vi "Telnet_test.vi"(5 "report_path":path, 6 "bytes to read (1024)":i32=1024, 7 "Delay Time (s)":dbl=0.3, 8 "error in (no error)":errorcluster, 9 "expected string":string, 10 "Command":string) -> (0 "error out":errorcluster, 1 "String found?":bool, 2 "string out":string caption="string ou", 3 "connection ID out":refnum<k5>)   [LabVIEW 2018]
doc: "This VI sends a command using telnet and verifies the response is the expected one."
panel:
  out "Get challenge status":string
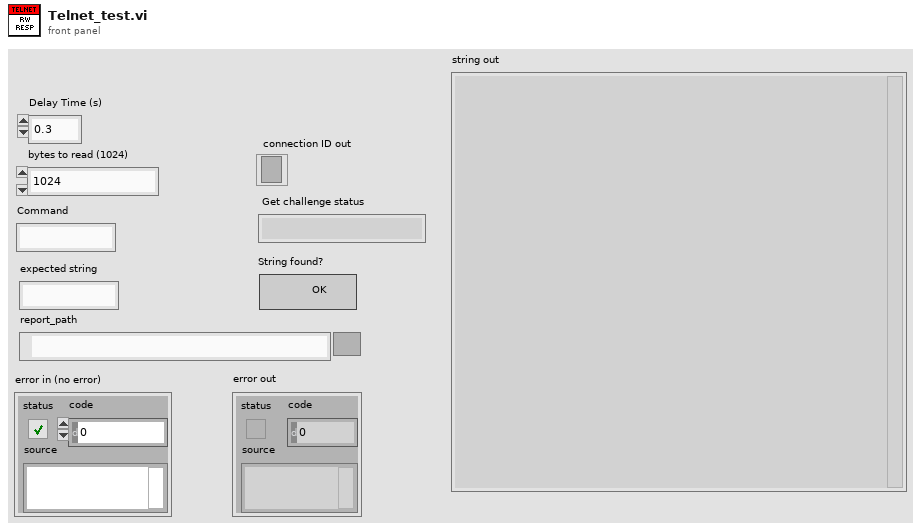
[diagram p1: front panel]
types:
  T1 = enum16{"Standard", "Buffered", "CRLF", "Immediate"}
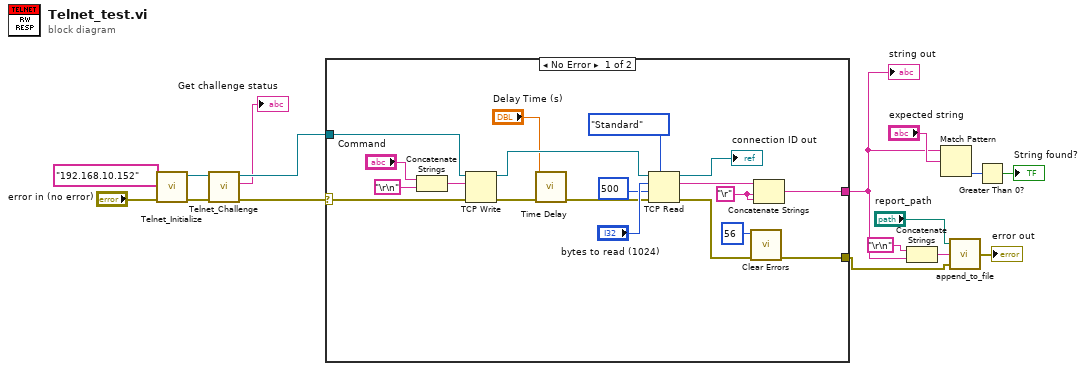
[diagram p0: block diagram]
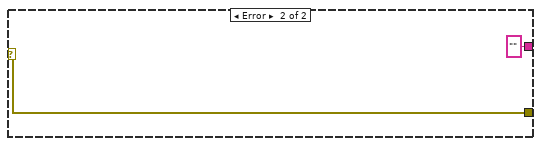
[diagram p2: hidden frame]
diagram:
  n1 = call "Telnet_Initialize.vi"("error in (no error)"="error in (no error)", "Address"="192.168.10.152") -> ("error out"=w5:errorcluster, "connection ID out"=w4:refnum<k5>)  [unwired: 8 in]
  n2 = call "Telnet_Challenge.vi"("error in (no error)"=w5, "connection ID in"=w4) -> ("error out"=w1:errorcluster, "Challenge status"=→"Get challenge status":string, "connection ID out"=w3:refnum<k5>)  [unwired: 7 in]
  n3 = case shown="No Error" w1 {
    selector: w1 -> [w19 w36]
    tunnel: [w26 ""] -> w9
    tunnel: [w25 w36] -> w8
    tunnel: w3 -> [w20 _]
    frame No Error {
      w27 = "\r"
      n4 = Concatenate Strings("Command", "\r\n") -> (w24:string)
      n5 = TCP Write(connection ID=w20, data in=w24, error in (no error)=w19) -> (connection ID out=w22:refnum<k5>, error out=w21:errorcluster)  [unwired: 1 in, 1 out]
      n6 = call "Time Delay"("error in (no error)"=w21, "Delay Time (s)"="Delay Time (s)") -> ("error out"=w29:errorcluster)  [unwired: 9 in]
      n7 = TCP Read(connection ID=w22, bytes to read="bytes to read (1024)", error in (no error)=w29, 7:T1."Standard" ("mode (standard)"), 9:500 ("timeout ms (25000)")) -> (connection ID out=→"connection ID out":refnum<k5>, data out=w28:string, error out=w32:errorcluster)
      n8 = call "Clear Errors.vi"("error in (no error)"=w32, "specific error code to clear (0: all)"=56) -> ("error out"=w25:errorcluster)  [unwired: 4 in, 1 out]
      n9 = Concatenate Strings(w28, w27, w27) -> (w26:string)
    }
    frame Error {
    }
  }
  "string out" <- w9
  n10 = Concatenate Strings("\r\n", w9) -> (w14:string)
  n11 = Match Pattern(string=w9, regular expression="expected string") -> (offset past match=w12:i32)  [unwired: 1 in, 3 out]
  n12 = call "append_to_file.vi"("error in (no error)"=w8, "text"=w14, "file_path"="report_path") -> ("error out"=→"error out":errorcluster)
  n13 = Greater Than 0?(x=w12) -> (x > 0?=→"String found?":bool)
